vi "FTW-Example-Service-Core-Initialize.vi"(0 "Initialization Sequence":string, 5 "FTW Actor Instance Configuration":string, 11 "error in (no error)":errorcluster) -> (4 "Actor Template-Core out":refnum<class "FTW-Example-Service-Core.lvclass">, 6 "Incoming Requests":refnum<event-registration>, 15 "error out":errorcluster)   [LabVIEW 2018, in "FTW-Example-Service-Core.lvclass"]
uses:
  FTW-Example-Service-Core.lvclass
  source/CodeGen/JSON Deserialize/FTW-JSON-Deserialize.xnode
  source/CodeGen/JSON Deserialize/FTW-JSON-Core-GetFlattenedValue.vi
  source/Reflection/FTW-Reflection-Type.vi
  source/JSON/core/FTW-JSON-Core-EncodingFlags.vi
  source/JSON/FTW-JSON-Parse.vi
  source/actor/Message/Request/FTW-Message-IncomingRequest.lvclass
  C:/Jobs/Featherweight/featherweight-2018/source/actor/Message/Base/FTW-Message.lvclass
  source/actor/Message/Base/FTW-Message.lvclass
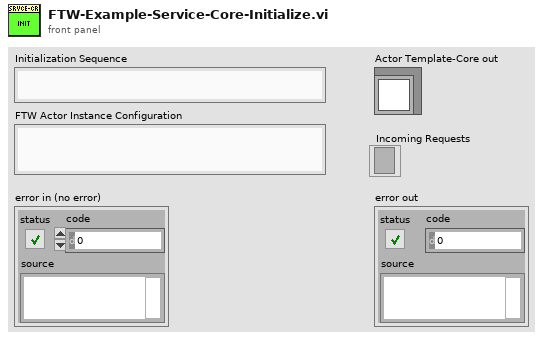
[diagram p1: front panel]
types:
  T1 = cluster{"Incoming Requests":refnum<event-registration>, "Local Messages":refnum<event-registration>, "Subscriber Registration":refnum<event-registration>}
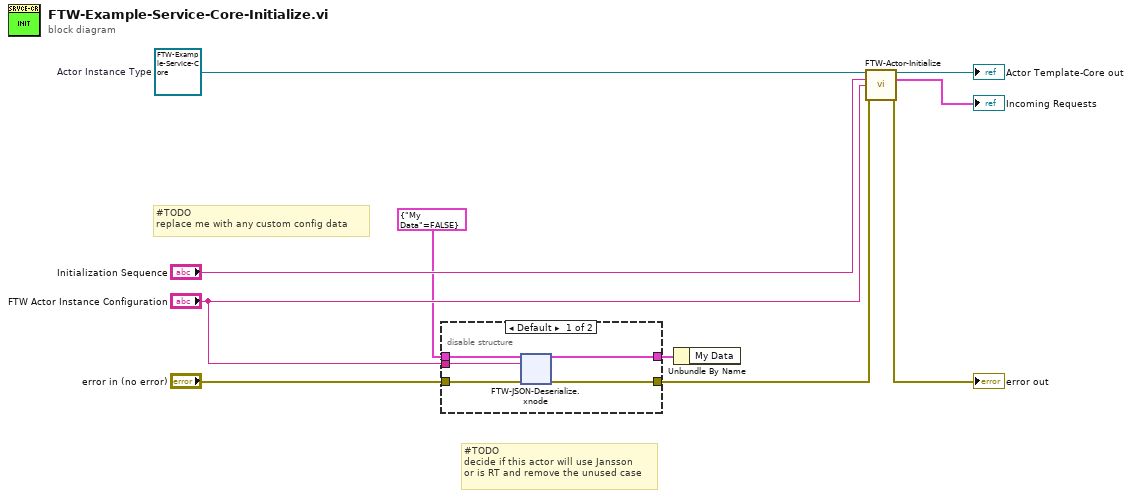
[diagram p0: block diagram]
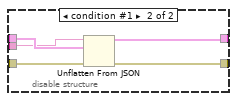
[diagram p2: hidden frame]
diagram:
  w1 = refnum<class "FTW-Example-Service-Core.lvclass"> refnum  # Actor Instance Type
  # "#TODO\ndecide if this actor will use Jansson\nor is RT and remove the unused case"
  # "#TODO\nreplace me with any custom config data"
  n1 = disable-structure shown="Default" {
    disable-tunnel: "error in (no error)" -> [w15 w32]
    disable-tunnel: [w14 w31] -> w5
    disable-tunnel: "FTW Actor Instance Configuration" -> [w13 w29]
    disable-tunnel: cluster{"My Data":bool} {"My Data"=FALSE} ("Type and Defaults") -> [w12 w30]
    disable-tunnel: [w11 w28] -> w2
    frame condition #0 (active) {
      n2 = xnode "FTW-JSON-Deserialize.xnode"("Type and Defaults"=w12, "JSON String"=w13, "error in"=w15) -> ("Values"=w11:cluster{"My Data":bool}, "error out"=w14:errorcluster)
    }
    frame condition #1 {
      n3 = Unflatten From JSON(JSON string=w29, type and defaults=w30, error in (no error)=w32) -> (value=w28:cluster{"My Data":bool}, error out=w31:errorcluster)  [unwired: 4 in]
    }
  }
  n4 = Unbundle By Name(w2) -> ()  [unwired: 1 out]
  n5 = call-dynamic "FTW-Actor-Initialize.vi"("FTW Actor Instance Type"=w1, "Initialization Job Sequence"="Initialization Sequence", "Actor Instance Configuration"="FTW Actor Instance Configuration", "error in"=w5) -> ("FTW Actor Instance"=→"Actor Template-Core out":refnum<class "FTW-Example-Service-Core.lvclass">, "Event Refnums"=→"Incoming Requests":T1, "error out"=→"error out":errorcluster)  [unwired: 9 in]
